vi "log analysis_gps.vi"() -> ()   [LabVIEW 2018] (continued)
126.72084266483,9.8311,22.3000,-0.0007,0.0064,0.0053,-0.805322808,0.199332071,80.524990625,0.2793,0.1938,0.4090,0.0347,0.0344,0.0317,0.0721,0.0737,4.9673,0f000005,0*f499bec4\n\tsystem status\texception 0 27.800000 0 32\trobot status\t0.669629\t-3.246177\t9.831100\t-0.805323\t0.199332\t9.475009\t0.147000\t0.222000\n\t\n15:54:09.0\tlog_raw\tgps_raw\t#INSPVAXA,USB3,0,45.0,FINESTEERING,2107,284067.050,02000000,471d,15824;INS_ALIGNMENT_COMPLETE,INS_RTKFIXED,37.37010094387,126.72084267852,9.8307,22.3000,-0.0007,0.0065,0.0059,-0.804077571,0.201412948,80.525848539,0.2693,0.1873,0.3960,0.0346,0.0343,0.0314,0.0722,0.0736,4.9532,0f000005,0*b106a646\n\tsystem status\texception 0 27.800000 0 32\trobot status\t0.670842\t-3.246592\t9.830700\t-0.804078\t0.201413\t9.474151\t0.147000\t0.222000\n\t\n15:54:09.5\tlog_raw\tgps_raw\t\tsystem status\texception 0 27.800000 0 32\trobot status\t0.671565\t-3.247256\t9.830100\t-0.803361\t0.201716\t9.474638\t0.147000\t0.222000\n\t\n15:54:10.0\tlog_raw\tgps_raw\t#INSPVAXA,USB3,0,45.0,FINESTEERING,2107,284068.050,02000000,471d,15824;INS_ALIGNMENT_COMPLETE,INS_RTKFIXED,37.37010093147,126.72084269859,9.8300,22.3000,-0.0011,0.0054,0.0061,-0.802134558,0.201672823,80.524962469,0.2605,0.1821,0.3846,0.0346,0.0343,0.0313,0.0723,0.0734,4.9387,0f000005,0*023ab06f\n\tsystem status\texception 0 27.800000 0 32\trobot status\t0.672620\t-3.247969\t9.830000\t-0.802135\t0.201673\t9.475038\t0.147000\t0.222000\n\t\n15:54:10.5\tlog_raw\tgps_raw\t\tsystem status\texception 0 27.800000 0 32\trobot status\t0.673184\t-3.248426\t9.829300\t-0.800656\t0.202458\t9.475344\t0.147000\t0.222000\n\t\n15:54:11.0\tlog_raw\tgps_raw\t\tsystem status\texception 0 27.800000 0 32\trobot status\t0.674167\t-3.248973\t9.829300\t-0.799789\t0.203840\t9.478232\t0.147000\t0.222000\n\t\n15:54:11.5\tlog_raw\tgps_raw\t#INSPVAXA,USB3,0,52.5,FINESTEERING,2107,284069.550,02000000,471d,15824;INS_ALIGNMENT_COMPLETE,INS_RTKFIXED,37.37010092244,126.72084272464,9.8293,22.3000,-0.0013,0.0057,0.0059,-0.798598974,0.203976276,80.516419675,0.2537,0.1782,0.3747,0.0345,0.0343,0.0313,0.0723,0.0733,4.9257,0f000005,0*56198093\n\tsystem status\texception 0 27.700000 0 32\trobot status\t0.674927\t-3.248971\t9.829300\t-0.798599\t0.203976\t9.483580\t0.147000\t0.222000\n\t\n15:54:12.0\tlog_raw\tgps_raw\t#INSPVAXA,USB3,0,52.5,FINESTEERING,2107,284070.050,02000000,471d,15824;INS_ALIGNMENT_COMPLETE,INS_RTKFIXED,37.37010091982,126.72084273744,9.8297,22.3000,-0.0012,0.0080,0.0052,-0.796727291,0.202371402,80.509450854,0.2478,0.1752,0.3659,0.0345,0.0343,0.0313,0.0724,0.0732,4.9128,0f000005,0*32eb7788\n\tsystem status\texception 0 27.800000 0 32\trobot status\t0.676061\t-3.249262\t9.829700\t-0.796727\t0.202371\t9.490549\t0.147000\t0.222000\n\t\n15:54:12.5\tlog_raw\tgps_raw\t\tsystem status\texception 0 27.800000 0 32\trobot status\t0.674655\t-3.249824\t9.829400\t-0.792783\t0.205130\t9.497173\t0.147000\t0.222000\n\t\n15:54:13.0\tlog_raw\tgps_raw\t#INSPVAXA,USB3,0,48.5,FINESTEERING,2107,284071.050,02000000,471d,15824;INS_ALIGNMENT_COMPLETE,INS_RTKFIXED,37.37010090434,126.72084271110,9.8295,22.3000,-0.0039,0.0026,0.0058,-0.794464008,0.206738241,80.502187928,0.2427,0.1727,0.3579,0.0345,0.0343,0.0313,0.0724,0.0732,4.9038,0f000005,0*ae7eb45b\n\tsystem status\texception 0 27.800000 0 32\trobot status\t0.673728\t-3.250980\t9.829500\t-0.794464\t0.206738\t9.497812\t0.147000\t0.222000\n\t\n15:54:13.5\tlog_raw\tgps_raw\t#INSPVAXA,USB3,0,48.5,FINESTEERING,2107,284071.550,02000000,471d,15824;INS_ALIGNMENT_COMPLETE,INS_RTKFIXED,37.37010089734,126.72084271003,9.8294,22.3000,-0.0047,0.0026,0.0048,-0.792309552,0.204330401,80.495522274,0.2427,0.1727,0.3579,0.0345,0.0343,0.0313,0.0724,0.0732,4.9038,0f000005,0*ad98db8e\n\tsystem status\texception 0 27.800000 0 32\trobot status\t0.673633\t-3.251756\t9.829400\t-0.792310\t0.204330\t9.504478\t0.147000\t0.222000\n\t\n15:54:14.0\tlog_raw\tgps_raw\t\tsystem status\texception 0 27.800000 0 32\trobot status\t0.673376\t-3.253810\t9.829800\t-0.795967\t0.184821\t9.359598\t0.117000\t0.095000\n\t\n15:54:14.5\tlog_raw\tgps_raw\t\tsystem status\texception 0 27.800000 0 60\trobot status\t0.674132\t-3.257605\t9.832900\t-0.788414\t0.193198\t9.387077\t0.117000\t0.095000\n\t\n15:54:15.0\tlog_raw\tgps_raw\t\tsystem status\texception 0 27.800000 0 60\trobot status\t0.676499\t-3.262353\t9.836500\t-0.786147\t0.194904\t9.385323\t0.117000\t0.095000\n\t\n15:54:15.5\tlog_raw\tgps_raw\t\tsystem status\texception 0 27.800000 0 60\trobot status\t0.678961\t-3.267673\t9.840700\t-0.786580\t0.194426\t9.385900\t0.117000\t0.095000\n\t\n15:54:16.0\tlog_raw\tgps_raw\t\tsystem status\texception 0 27.800000 0 60\trobot status\t0.682045\t-3.274174\t9.845300\t-0.785139\t0.194086\t9.384595\t0.117000\t0.095000\n\t\n15:54:16.5\tlog_raw\tgps_raw\t\tsystem status\texception 0 27.800000 0 60\trobot status\t0.684298\t-3.281012\t9.849500\t-0.785110\t0.192293\t9.376254\t0.117000\t0.095000\n\t\n15:54:17.0\tlog_raw\tgps_raw\t\tsystem status\texception 0 27.800000 0 60\trobot status\t0.687811\t-3.288802\t9.854200\t-0.783660\t0.192337\t9.377009\t0.117000\t0.095000\n\t\n15:54:17.5\tlog_raw\tgps_raw\t\tsystem status\texception 0 27.800000 0 60\trobot status\t0.690737\t-3.295775\t9.858800\t-0.784560\t0.190680\t9.377608\t0.117000\t0.095000\n\t\n15:54:18.0\tlog_raw\tgps_raw\t#INSPVAXA,USB3,0,53.5,FINESTEERING,2107,284076.050,02000000,471d,15824;INS_ALIGNMENT_COMPLETE,INS_RTKFIXED,37.37010043153,126.72084293702,9.8639,22.3000,-0.0224,0.0084,0.0124,-0.782520442,0.190697298,80.620510756,0.3079,0.2467,0.3912,0.0928,0.0849,0.0629,0.0895,0.0915,4.9091,0f000001,0*151fdb37\n\tsystem status\texception 0 27.800000 0 60\trobot status\t0.693740\t-3.303454\t9.863900\t-0.782520\t0.190697\t9.379489\t0.117000\t0.095000\n\t\n15:54:18.5\tlog_raw\tgps_raw\t\tsystem status\texception 0 27.800000 0 60\trobot status\t0.697678\t-3.308999\t9.869500\t-0.783353\t0.190598\t9.384457\t0.117000\t0.095000\n\t\n15:54:19.0\tlog_raw\tgps_raw\t\tsystem status\texception 0 27.800000 0 60\trobot status\t0.701548\t-3.315091\t9.875400\t-0.783389\t0.191366\t9.388017\t0.117000\t0.095000\n\t\n15:54:19.5\tlog_raw\tgps_raw\t#INSPVAXA,USB3,0,53.0,FINESTEERING,2107,284077.550,02000000,471d,15824;INS_ALIGNMENT_COMPLETE,INS_RTKFIXED,37.37010029205,126.72084303769,9.8807,22.3000,-0.0245,0.0085,0.0134,-0.783196665,0.189878552,80.605229248,0.3387,0.2662,0.4111,0.1003,0.0889,0.0668,0.0907,0.0935,4.9083,0f000001,0*a805bdc6\n\tsystem status\texception 0 27.800000 0 60\trobot status\t0.702657\t-3.318934\t9.880700\t-0.783197\t0.189879\t9.394771\t0.117000\t0.095000\n\t\n15:54:20.0\tlog_raw\tgps_raw\t\t", "INSPVAXA,USB3,0,52.0,FINESTEERING,2107,284098.100,02000000,471d,15824;INS_ALIGNMENT_COMPLETE,INS_RTKFIXED,37.37010081715,126.72084280567,9.8392,22.3000,-0.0127,0.0026,0.0011,-0.779185291,0.204850370,80.324830339,0.2135,0.1621,0.2919,0.0344,0.0343,0.0312,0.0727,0.0733,4.8847,0f000005,0*b965a086\n\t", "INSPVAXA,USB3,0,53.0,FINESTEERING,2107,284099.100,02000000,471d,15824;INS_ALIGNMENT_COMPLETE,INS_RTKFIXED,37.37010080039,126.72084280580,9.8388,22.3000,-0.0144,0.0013,0.0007,-0.778559962,0.207012458,80.310324133,0.2130,0.1619,0.2904,0.0344,0.0343,0.0312,0.0727,0.0733,4.8855,0f000005,0*91b9a8e7\n\t", "INSPVAXA,USB3,0,50.0,FINESTEERING,2107,284101.100,02000000,471d,15824;INS_ALIGNMENT_COMPLETE,INS_RTKFIXED,37.37010080256,126.72084279427,9.8376,22.3000,-0.0100,0.0003,0.0004,-0.784971071,0.210053203,80.284000785,0.2120,0.1618,0.2876,0.0344,0.0343,0.0312,0.0727,0.0733,4.8873,0f000005,0*ce207b7d\n\t", "INSPVAXA,USB3,0,50.0,FINESTEERING,2107,284101.600,02000000,471d,15824;INS_ALIGNMENT_COMPLETE,INS_RTKFIXED,37.37010080771,126.72084279588,9.8375,22.3000,-0.0097,0.0008,0.0002,-0.787245577,0.212021074,80.277840242,0.2120,0.1618,0.2876,0.0344,0.0343,0.0312,0.0727,0.0733,4.8873,0f000005,0*d3394abe\n\t", "INSPVAXA,USB3,0,53.0,FINESTEERING,2107,284102.100,02000000,471d,15824;INS_ALIGNMENT_COMPLETE,INS_RTKFIXED,37.37010080827,126.72084279791,9.8372,22.3000,-0.0086,0.0007,-0.0005,-0.787222200,0.211318071,80.272885297,0.2116,0.1617,0.2864,0.0344,0.0343,0.0312,0.0727,0.0733,4.8883,0f000005,0*7e8ab6e8\n\t", "INSPVAXA,USB3,0,53.0,FINESTEERING,2107,284103.100,02000000,471d,15824;INS_ALIGNMENT_COMPLETE,INS_RTKFIXED,37.37010082403,126.72084278484,9.8365,22.3000,-0.0064,-0.0008,-0.0001,-0.787428816,0.215864037,80.263823554,0.2112,0.1616,0.2853,0.0344,0.0343,0.0312,0.0727,0.0733,4.8894,0f000005,0*f475c441\n\t", "INSPVAXA,USB3,0,53.0,FINESTEERING,2107,284104.050,02000000,471d,15824;INS_ALIGNMENT_COMPLETE,INS_RTKFIXED,37.37010082408,126.72084278410,9.8363,22.3000,-0.0077,0.0002,0.0002,-0.786930858,0.220983047,80.255496235,0.2109,0.1616,0.2842,0.0344,0.0343,0.0312,0.0727,0.0733,4.8905,0f000005,0*84218c18\n\t", "INSPVAXA,USB3,0,53.0,FINESTEERING,2107,284104.050,02000000,471d,15824;INS_ALIGNMENT_COMPLETE,INS_RTKFIXED,37.37010082408,126.72084278410,9.8363,22.3000,-0.0077,0.0002,0.0002,-0.786930858,0.220983047,80.255496235,0.2109,0.1616,0.2842,0.0344,0.0343,0.0312,0.0727,0.0733,4.8905,0f000005,0*84218c18\n\t", "INSPVAXA,USB3,0,53.0,FINESTEERING,2107,284104.050,02000000,471d,15824;INS_ALIGNMENT_COMPLETE,INS_RTKFIXED,37.37010082408,126.72084278410,9.8363,22.3000,-0.0077,0.0002,0.0002,-0.786930858,0.220983047,80.255496235,0.2109,0.1616,0.2842,0.0344,0.0343,0.0312,0.0727,0.0733,4.8905,0f000005,0*84218c18\n\t", "INSPVAXA,USB3,0,53.0,FINESTEERING,2107,284104.050,02000000,471d,15824;INS_ALIGNMENT_COMPLETE,INS_RTKFIXED,37.37010082408,126.72084278410,9.8363,22.3000,-0.0077,0.0002,0.0002,-0.786930858,0.220983047,80.255496235,0.2109,0.1616,0.2842,0.0344,0.0343,0.0312,0.0727,0.0733,4.8905,0f000005,0*84218c18\n\t", "INSPVAXA,USB3,0,53.0,FINESTEERING,2107,284104.050,02000000,471d,15824;INS_ALIGNMENT_COMPLETE,INS_RTKFIXED,37.37010082408,126.72084278410,9.8363,22.3000,-0.0077,0.0002,0.0002,-0.786930858,0.220983047,80.255496235,0.2109,0.1616,0.2842,0.0344,0.0343,0.0312,0.0727,0.0733,4.8905,0f000005,0*84218c18\n\t", "INSPVAXA,USB3,0,53.0,FINESTEERING,2107,284104.050,02000000,471d,15824;INS_ALIGNMENT_COMPLETE,INS_RTKFIXED,37.37010082408,126.72084278410,9.8363,22.3000,-0.0077,0.0002,0.0002,-0.786930858,0.220983047,80.255496235,0.2109,0.1616,0.2842,0.0344,0.0343,0.0312,0.0727,0.0733,4.8905,0f000005,0*84218c18\n\t", "INSPVAXA,USB3,0,53.0,FINESTEERING,2107,284104.050,02000000,471d,15824;INS_ALIGNMENT_COMPLETE,INS_RTKFIXED,37.37010082408,126.72084278410,9.8363,22.3000,-0.0077,0.0002,0.0002,-0.786930858,0.220983047,80.255496235,0.2109,0.1616,0.2842,0.0344,0.0343,0.0312,0.0727,0.0733,4.8905,0f000005,0*84218c18\n\t", "INSPVAXA,USB3,0,53.0,FINESTEERING,2107,284104.050,02000000,471d,15824;INS_ALIGNMENT_COMPLETE,INS_RTKFIXED,37.37010082408,126.72084278410,9.8363,22.3000,-0.0077,0.0002,0.0002,-0.786930858,0.220983047,80.255496235,0.2109,0.1616,0.2842,0.0344,0.0343,0.0312,0.0727,0.0733,4.8905,0f000005,0*84218c18\n\t", "INSPVAXA,USB3,0,53.0,FINESTEERING,2107,284104.050,02000000,471d,15824;INS_ALIGNMENT_COMPLETE,INS_RTKFIXED,37.37010082408,126.72084278410,9.8363,22.3000,-0.0077,0.0002,0.0002,-0.786930858,0.220983047,80.255496235,0.2109,0.1616,0.2842,0.0344,0.0343,0.0312,0.0727,0.0733,4.8905,0f000005,0*84218c18\n\t", "INSPVAXA,USB3,0,53.0,FINESTEERING,2107,284104.050,02000000,471d,15824;INS_ALIGNMENT_COMPLETE,INS_RTKFIXED,37.37010082408,126.72084278410,9.8363,22.3000,-0.0077,0.0002,0.0002,-0.786930858,0.220983047,80.255496235,0.2109,0.1616,0.2842,0.0344,0.0343,0.0312,0.0727,0.0733,4.8905,0f000005,0*84218c18\n\t", "INSPVAXA,USB3,0,53.0,FINESTEERING,2107,284104.050,02000000,471d,15824;INS_ALIGNMENT_COMPLETE,INS_RTKFIXED,37.37010082408,126.72084278410,9.8363,22.3000,-0.0077,0.0002,0.0002,-0.786930858,0.220983047,80.255496235,0.2109,0.1616,0.2842,0.0344,0.0343,0.0312,0.0727,0.0733,4.8905,0f000005,0*84218c18\n\t", "INSPVAXA,USB3,0,53.0,FINESTEERING,2107,284104.050,02000000,471d,15824;INS_ALIGNMENT_COMPLETE,INS_RTKFIXED,37.37010082408,126.72084278410,9.8363,22.3000,-0.0077,0.0002,0.0002,-0.786930858,0.220983047,80.255496235,0.2109,0.1616,0.2842,0.0344,0.0343,0.0312,0.0727,0.0733,4.8905,0f000005,0*84218c18\n\t", "INSPVAXA,USB3,0,53.0,FINESTEERING,2107,284104.050,02000000,471d,15824;INS_ALIGNMENT_COMPLETE,INS_RTKFIXED,37.37010082408,126.72084278410,9.8363,22.3000,-0.0077,0.0002,0.0002,-0.786930858,0.220983047,80.255496235,0.2109,0.1616,0.2842,0.0344,0.0343,0.0312,0.0727,0.0733,4.8905,0f000005,0*84218c18\n\t", "INSPVAXA,USB3,0,53.0,FINESTEERING,2107,284104.050,02000000,471d,15824;INS_ALIGNMENT_COMPLETE,INS_RTKFIXED,37.37010082408,126.72084278410,9.8363,22.3000,-0.0077,0.0002,0.0002,-0.786930858,0.220983047,80.255496235,0.2109,0.1616,0.2842,0.0344,0.0343,0.0312,0.0727,0.0733,4.8905,0f000005,0*84218c18\n\t", "INSPVAXA,USB3,0,53.0,FINESTEERING,2107,284104.050,02000000,471d,15824;INS_ALIGNMENT_COMPLETE,INS_RTKFIXED,37.37010082408,126.72084278410,9.8363,22.3000,-0.0077,0.0002,0.0002,-0.786930858,0.220983047,80.255496235,0.2109,0.1616,0.2842,0.0344,0.0343,0.0312,0.0727,0.0733,4.8905,0f000005,0*84218c18\n\t", "INSPVAXA,USB3,0,53.0,FINESTEERING,2107,284104.050,02000000,471d,15824;INS_ALIGNMENT_COMPLETE,INS_RTKFIXED,37.37010082408,126.72084278410,9.8363,22.3000,-0.0077,0.0002,0.0002,-0.786930858,0.220983047,80.255496235,0.2109,0.1616,0.2842,0.0344,0.0343,0.0312,0.0727,0.0733,4.8905,0f000005,0*84218c18\n\t", "INSPVAXA,USB3,0,53.0,FINESTEERING,2107,284104.050,02000000,471d,15824;INS_ALIGNMENT_COMPLETE,INS_RTKFIXED,37.37010082408,126.72084278410,9.8363,22.3000,-0.0077,0.0002,0.0002,-0.786930858,0.220983047,80.255496235,0.2109,0.1616,0.2842,0.0344,0.0343,0.0312,0.0727,0.0733,4.8905,0f000005,0*84218c18\n\t", "INSPVAXA,USB3,0,53.0,FINESTEERING,2107,284104.050,02000000,471d,15824;INS_ALIGNMENT_COMPLETE,INS_RTKFIXED,37.37010082408,126.72084278410,9.8363,22.3000,-0.0077,0.0002,0.0002,-0.786930858,0.220983047,80.255496235,0.2109,0.1616,0.2842,0.0344,0.0343,0.0312,0.0727,0.0733,4.8905,0f000005,0*84218c18\n\t", "INSPVAXA,USB3,0,53.0,FINESTEERING,2107,284104.050,02000000,471d,15824;INS_ALIGNMENT_COMPLETE,INS_RTKFIXED,37.37010082408,126.72084278410,9.8363,22.3000,-0.0077,0.0002,0.0002,-0.786930858,0.220983047,80.255496235,0.2109,0.1616,0.2842,0.0344,0.0343,0.0312,0.0727,0.0733,4.8905,0f000005,0*84218c18\n\t", "INSPVAXA,USB3,0,53.0,FINESTEERING,2107,284104.050,02000000,471d,15824;INS_ALIGNMENT_COMPLETE,INS_RTKFIXED,37.37010082408,126.72084278410,9.8363,22.3000,-0.0077,0.0002,0.0002,-0.786930858,0.220983047,80.255496235,0.2109,0.1616,0.2842,0.0344,0.0343,0.0312,0.0727,0.0733,4.8905,0f000005,0*84218c18\n\t", "INSPVAXA,USB3,0,53.0,FINESTEERING,2107,284104.050,02000000,471d,15824;INS_ALIGNMENT_COMPLETE,INS_RTKFIXED,37.37010082408,126.72084278410,9.8363,22.3000,-0.0077,0.0002,0.0002,-0.786930858,0.220983047,80.255496235,0.2109,0.1616,0.2842,0.0344,0.0343,0.0312,0.0727,0.0733,4.8905,0f000005,0*84218c18\n\t", "INSPVAXA,USB3,0,53.0,FINESTEERING,2107,284104.050,02000000,471d,15824;INS_ALIGNMENT_COMPLETE,INS_RTKFIXED,37.37010082408,126.72084278410,9.8363,22.3000,-0.0077,0.0002,0.0002,-0.786930858,0.220983047,80.255496235,0.2109,0.1616,0.2842,0.0344,0.0343,0.0312,0.0727,0.0733,4.8905,0f000005,0*84218c18\n\t", "INSPVAXA,USB3,0,53.0,FINESTEERING,2107,284104.050,02000000,471d,15824;INS_ALIGNMENT_COMPLETE,INS_RTKFIXED,37.37010082408,126.72084278410,9.8363,22.3000,-0.0077,0.0002,0.0002,-0.786930858,0.220983047,80.255496235,0.2109,0.1616,0.2842,0.0344,0.0343,0.0312,0.0727,0.0733,4.8905,0f000005,0*84218c18\n\t", "INSPVAXA,USB3,0,53.0,FINESTEERING,2107,284104.050,02000000,471d,15824;INS_ALIGNMENT_COMPLETE,INS_RTKFIXED,37.37010082408,126.72084278410,9.8363,22.3000,-0.0077,0.0002,0.0002,-0.786930858,0.220983047,80.255496235,0.2109,0.1616,0.2842,0.0344,0.0343,0.0312,0.0727,0.0733,4.8905,0f000005,0*84218c18\n\t", "INSPVAXA,USB3,0,53.0,FINESTEERING,2107,284104.050,02000000,471d,15824;INS_ALIGNMENT_COMPLETE,INS_RTKFIXED,37.37010082408,126.72084278410,9.8363,22.3000,-0.0077,0.0002,0.0002,-0.786930858,0.220983047,80.255496235,0.2109,0.1616,0.2842,0.0344,0.0343,0.0312,0.0727,0.0733,4.8905,0f000005,0*84218c18\n\t", "INSPVAXA,USB3,0,53.0,FINESTEERING,2107,284104.050,02000000,471d,15824;INS_ALIGNMENT_COMPLETE,INS_RTKFIXED,37.37010082408,126.72084278410,9.8363,22.3000,-0.0077,0.0002,0.0002,-0.786930858,0.220983047,80.255496235,0.2109,0.1616,0.2842,0.0344,0.0343,0.0312,0.0727,0.0733,4.8905,0f000005,0*84218c18\n\t", "INSPVAXA,USB3,0,53.0,FINESTEERING,2107,284104.050,02000000,471d,15824;INS_ALIGNMENT_COMPLETE,INS_RTKFIXED,37.37010082408,126.72084278410,9.8363,22.3000,-0.0077,0.0002,0.0002,-0.786930858,0.220983047,80.255496235,0.2109,0.1616,0.2842,0.0344,0.0343,0.0312,0.0727,0.0733,4.8905,0f000005,0*84218c18\n\t", "INSPVAXA,USB3,0,53.0,FINESTEERING,2107,284104.050,02000000,471d,15824;INS_ALIGNMENT_COMPLETE,INS_RTKFIXED,37.37010082408,126.72084278410,9.8363,22.3000,-0.0077,0.0002,0.0002,-0.786930858,0.220983047,80.255496235,0.2109,0.1616,0.2842,0.0344,0.0343,0.0312,0.0727,0.0733,4.8905,0f000005,0*84218c18\n\t", "INSPVAXA,USB3,0,53.0,FINESTEERING,2107,284104.050,02000000,471d,15824;INS_ALIGNMENT_COMPLETE,INS_RTKFIXED,37.37010082408,126.72084278410,9.8363,22.3000,-0.0077,0.0002,0.0002,-0.786930858,0.220983047,80.255496235,0.2109,0.1616,0.2842,0.0344,0.0343,0.0312,0.0727,0.0733,4.8905,0f000005,0*84218c18\n\t", "INSPVAXA,USB3,0,53.0,FINESTEERING,2107,284104.050,02000000,471d,15824;INS_ALIGNMENT_COMPLETE,INS_RTKFIXED,37.37010082408,126.72084278410,9.8363,22.3000,-0.0077,0.0002,0.0002,-0.786930858,0.220983047,80.255496235,0.2109,0.1616,0.2842,0.0344,0.0343,0.0312,0.0727,0.0733,4.8905,0f000005,0*84218c18\n\t", "INSPVAXA,USB3,0,53.0,FINESTEERING,2107,284104.050,02000000,471d,15824;INS_ALIGNMENT_COMPLETE,INS_RTKFIXED,37.37010082408,126.72084278410,9.8363,22.3000,-0.0077,0.0002,0.0002,-0.786930858,0.220983047,80.255496235,0.2109,0.1616,0.2842,0.0344,0.0343,0.0312,0.0727,0.0733,4.8905,0f000005,0*84218c18\n\t", "INSPVAXA,USB3,0,53.0,FINESTEERING,2107,284104.050,02000000,471d,15824;INS_ALIGNMENT_COMPLETE,INS_RTKFIXED,37.37010082408,126.72084278410,9.8363,22.3000,-0.0077,0.0002,0.0002,-0.786930858,0.220983047,80.255496235,0.2109,0.1616,0.2842,0.0344,0.0343,0.0312,0.0727,0.0733,4.8905,0f000005,0*84218c18\n\t", "INSPVAXA,USB3,0,53.0,FINESTEERING,2107,284104.050,02000000,471d,15824;INS_ALIGNMENT_COMPLETE,INS_RTKFIXED,37.37010082408,126.72084278410,9.8363,22.3000,-0.0077,0.0002,0.0002,-0.786930858,0.220983047,80.255496235,0.2109,0.1616,0.2842,0.0344,0.0343,0.0312,0.0727,0.0733,4.8905,0f000005,0*84218c18\n\t", "INSPVAXA,USB3,0,53.0,FINESTEERING,2107,284104.050,02000000,471d,15824;INS_ALIGNMENT_COMPLETE,INS_RTKFIXED,37.37010082408,126.72084278410,9.8363,22.3000,-0.0077,0.0002,0.0002,-0.786930858,0.220983047,80.255496235,0.2109,0.1616,0.2842,0.0344,0.0343,0.0312,0.0727,0.0733,4.8905,0f000005,0*84218c18\n\t", "INSPVAXA,USB3,0,53.0,FINESTEERING,2107,284104.050,02000000,471d,15824;INS_ALIGNMENT_COMPLETE,INS_RTKFIXED,37.37010082408,126.72084278410,9.8363,22.3000,-0.0077,0.0002,0.0002,-0.786930858,0.220983047,80.255496235,0.2109,0.1616,0.2842,0.0344,0.0343,0.0312,0.0727,0.0733,4.8905,0f000005,0*84218c18\n\t", "INSPVAXA,USB3,0,53.0,FINESTEERING,2107,284104.050,02000000,471d,15824;INS_ALIGNMENT_COMPLETE,INS_RTKFIXED,37.37010082408,126.72084278410,9.8363,22.3000,-0.0077,0.0002,0.0002,-0.786930858,0.220983047,80.255496235,0.2109,0.1616,0.2842,0.0344,0.0343,0.0312,0.0727,0.0733,4.8905,0f000005,0*84218c18\n\t", "INSPVAXA,USB3,0,53.0,FINESTEERING,2107,284104.050,02000000,471d,15824;INS_ALIGNMENT_COMPLETE,INS_RTKFIXED,37.37010082408,126.72084278410,9.8363,22.3000,-0.0077,0.0002,0.0002,-0.786930858,0.220983047,80.255496235,0.2109,0.1616,0.2842,0.0344,0.0343,0.0312,0.0727,0.0733,4.8905,0f000005,0*84218c18\n\t", "INSPVAXA,USB3,0,53.0,FINESTEERING,2107,284104.050,02000000,471d,15824;INS_ALIGNMENT_COMPLETE,INS_RTKFIXED,37.37010082408,126.72084278410,9.8363,22.3000,-0.0077,0.0002,0.0002,-0.786930858,0.220983047,80.255496235,0.2109,0.1616,0.2842,0.0344,0.0343,0.0312,0.0727,0.0733,4.8905,0f000005,0*84218c18\n\t", "INSPVAXA,USB3,0,53.0,FINESTEERING,2107,284104.050,02000000,471d,15824;INS_ALIGNMENT_COMPLETE,INS_RTKFIXED,37.37010082408,126.72084278410,9.8363,22.3000,-0.0077,0.0002,0.0002,-0.786930858,0.220983047,80.255496235,0.2109,0.1616,0.2842,0.0344,0.0343,0.0312,0.0727,0.0733,4.8905,0f000005,0*84218c18\n\t", "INSPVAXA,USB3,0,53.0,FINESTEERING,2107,284104.050,02000000,471d,15824;INS_ALIGNMENT_COMPLETE,INS_RTKFIXED,37.37010082408,126.72084278410,9.8363,22.3000,-0.0077,0.0002,0.0002,-0.786930858,0.220983047,80.255496235,0.2109,0.1616,0.2842,0.0344,0.0343,0.0312,0.0727,0.0733,4.8905,0f000005,0*84218c18\n\t", "INSPVAXA,USB3,0,53.0,FINESTEERING,2107,284104.050,02000000,471d,15824;INS_ALIGNMENT_COMPLETE,INS_RTKFIXED,37.37010082408,126.72084278410,9.8363,22.3000,-0.0077,0.0002,0.0002,-0.786930858,0.220983047,80.255496235,0.2109,0.1616,0.2842,0.0344,0.0343,0.0312,0.0727,0.0733,4.8905,0f000005,0*84218c18\n\t", "INSPVAXA,USB3,0,53.0,FINESTEERING,2107,284104.050,02000000,471d,15824;INS_ALIGNMENT_COMPLETE,INS_RTKFIXED,37.37010082408,126.72084278410,9.8363,22.3000,-0.0077,0.0002,0.0002,-0.786930858,0.220983047,80.255496235,0.2109,0.1616,0.2842,0.0344,0.0343,0.0312,0.0727,0.0733,4.8905,0f000005,0*84218c18\n\t", "INSPVAXA,USB3,0,53.0,FINESTEERING,2107,284104.050,02000000,471d,15824;INS_ALIGNMENT_COMPLETE,INS_RTKFIXED,37.37010082408,126.72084278410,9.8363,22.3000,-0.0077,0.0002,0.0002,-0.786930858,0.220983047,80.255496235,0.2109,0.1616,0.2842,0.0344,0.0343,0.0312,0.0727,0.0733,4.8905,0f000005,0*84218c18\n\t", "INSPVAXA,USB3,0,53.0,FINESTEERING,2107,284104.050,02000000,471d,15824;INS_ALIGNMENT_COMPLETE,INS_RTKFIXED,37.37010082408,126.72084278410,9.8363,22.3000,-0.0077,0.0002,0.0002,-0.786930858,0.220983047,80.255496235,0.2109,0.1616,0.2842,0.0344,0.0343,0.0312,0.0727,0.0733,4.8905,0f000005,0*84218c18\n\t", "INSPVAXA,USB3,0,53.0,FINESTEERING,2107,284104.050,02000000,471d,15824;INS_ALIGNMENT_COMPLETE,INS_RTKFIXED,37.37010082408,126.72084278410,9.8363,22.3000,-0.0077,0.0002,0.0002,-0.786930858,0.220983047,80.255496235,0.2109,0.1616,0.2842,0.0344,0.0343,0.0312,0.0727,0.0733,4.8905,0f000005,0*84218c18\n\t", "INSPVAXA,USB3,0,53.0,FINESTEERING,2107,284104.050,02000000,471d,15824;INS_ALIGNMENT_COMPLETE,INS_RTKFIXED,37.37010082408,126.72084278410,9.8363,22.3000,-0.0077,0.0002,0.0002,-0.786930858,0.220983047,80.255496235,0.2109,0.1616,0.2842,0.0344,0.0343,0.0312,0.0727,0.0733,4.8905,0f000005,0*84218c18\n\t", "INSPVAXA,USB3,0,53.0,FINESTEERING,2107,284104.050,02000000,471d,15824;INS_ALIGNMENT_COMPLETE,INS_RTKFIXED,37.37010082408,126.72084278410,9.8363,22.3000,-0.0077,0.0002,0.0002,-0.786930858,0.220983047,80.255496235,0.2109,0.1616,0.2842,0.0344,0.0343,0.0312,0.0727,0.0733,4.8905,0f000005,0*84218c18\n\t", "INSPVAXA,USB3,0,53.0,FINESTEERING,2107,284104.050,02000000,471d,15824;INS_ALIGNMENT_COMPLETE,INS_RTKFIXED,37.37010082408,126.72084278410,9.8363,22.3000,-0.0077,0.0002,0.0002,-0.786930858,0.220983047,80.255496235,0.2109,0.1616,0.2842,0.0344,0.0343,0.0312,0.0727,0.0733,4.8905,0f000005,0*84218c18\n\t", "INSPVAXA,USB3,0,53.0,FINESTEERING,2107,284104.050,02000000,471d,15824;INS_ALIGNMENT_COMPLETE,INS_RTKFIXED,37.37010082408,126.72084278410,9.8363,22.3000,-0.0077,0.0002,0.0002,-0.786930858,0.220983047,80.255496235,0.2109,0.1616,0.2842,0.0344,0.0343,0.0312,0.0727,0.0733,4.8905,0f000005,0*84218c18\n\t", "INSPVAXA,USB3,0,53.0,FINESTEERING,2107,284104.050,02000000,471d,15824;INS_ALIGNMENT_COMPLETE,INS_RTKFIXED,37.37010082408,126.72084278410,9.8363,22.3000,-0.0077,0.0002,0.0002,-0.786930858,0.220983047,80.255496235,0.2109,0.1616,0.2842,0.0344,0.0343,0.0312,0.0727,0.0733,4.8905,0f000005,0*84218c18\n\t", ""]
  out "이전 부분 문자열":string
  in  "load":bool
  in  "path":path=path "C:/Users/WeGo/Desktop/patrol robot/log/patrol-0527_log.txt"
  out "텍스트":string="15:04:55.6\tlog_raw\tgps_raw\t\tsystem status\tnormal 0 28.400000 0 0\trobot status\t0.573944\t0.974098\t9.870700\t-0.040116\t-0.068991\t52.206776\t0.000000\t-0.001000\n\t\n15:04:56.1\tlog_raw\tgps_raw\t\tsystem status\tnormal 0 28.400000 0 0\trobot status\t0.573944\t0.974098\t9.870700\t-0.040116\t-0.068991\t52.206776\t0.000000\t-0.001000\n\t\n15:04:56.6\tlog_raw\tgps_raw\t\tsystem status\tnormal 0 28.400000 0 0\trobot status\t0.573944\t0.974098\t9.870700\t-0.040116\t-0.068991\t52.206776\t0.000000\t-0.001000\n\t\n15:04:57.1\tlog_raw\tgps_raw\t\tsystem status\tnormal 0 28.400000 0 0\trobot status\t0.573944\t0.974098\t9.870700\t-0.040116\t-0.068991\t52.206776\t0.000000\t-0.001000\n\t\n15:04:57.6\tlog_raw\tgps_raw\t\tsystem status\tnormal 0 28.400000 0 0\trobot status\t0.573944\t0.974098\t9.870700\t-0.040116\t-0.068991\t52.206776\t0.000000\t-0.001000\n\t\n15:04:58.1\tlog_raw\tgps_raw\t\tsystem status\tnormal 0 28.400000 0 0\trobot status\t0.573944\t0.974098\t9.870700\t-0.040116\t-0.068991\t52.206776\t0.000000\t-0.001000\n\t\n15:04:58.6\tlog_raw\tgps_raw\t\tsystem status\tnormal 0 28.300000 0 0\trobot status\t0.573944\t0.974098\t9.870700\t-0.040116\t-0.068991\t52.206776\t0.000000\t-0.001000\n\t\n15:04:59.1\tlog_raw\tgps_raw\t\tsystem status\tnormal 0 28.400000 0 0\trobot status\t0.573944\t0.974098\t9.870700\t-0.040116\t-0.068991\t52.206776\t0.000000\t-0.001000\n\t\n15:04:59.6\tlog_raw\tgps_raw\t\tsystem status\tnormal 0 28.400000 0 0\trobot status\t0.573944\t0.974098\t9.870700\t-0.040116\t-0.068991\t52.206776\t0.000000\t-0.001000\n\t\n15:05:00.1\tlog_raw\tgps_raw\t#INSPVAXA,USB3,0,51.0,FINESTEERING,2107,281115.600,02000000,471d,15824;INS_ALIGNMENT_COMPLETE,INS_RTKFIXED,37.37013888668,126.72084169564,9.8834,22.3000,0.0026,0.0071,0.0017,-0.044376618,-0.064379115,35.875304095,0.1980,0.1670,0.2645,0.0373,0.0373,0.0312,0.3280,0.3375,5.4270,0f000015,0*6411398e\n\tsystem status\tnormal 0 28.400000 0 0\trobot status\t0.583780\t0.964475\t9.883400\t-0.044377\t-0.064379\t52.206776\t0.000000\t-0.001000\n\t\n15:05:00.6\tlog_raw\tgps_raw\t#DUALANTENNAHEADINGA,USB3,0,47.5,FINESTEERING,2107,281116.400,02000000,d426,15824;SOL_COMPUTED,NARROW_INT,-1.000000000,37.878738403,-13.522033691,0.0,0.725115359,0.922636747,\"631T\",26,18,18,14,04,01,30,33*26208e7b\n\tsystem status\tnormal 0 28.400000 0 0\trobot status\t0.584352\t0.964624\t9.883500\t-0.048962\t-0.060425\t52.121262\t0.000000\t0.000000\n\t\n15:05:01.1\tlog_raw\tgps_raw\t#INSPVAXA,USB3,0,40.0,FINESTEERING,2107,281117.200,02000000,471d,15824;INS_ALIGNMENT_COMPLETE,INS_RTKFIXED,37.37013888274,126.72084170690,9.8836,22.3000,0.0013,0.0059,0.0019,-0.052026954,-0.057051348,35.889318154,0.1981,0.1668,0.2641,0.0380,0.0379,0.0312,0.3290,0.3384,5.4011,0f000015,0*fd51250c\n\tsystem status\tnormal 0 28.400000 0 0\trobot status\t0.584778\t0.964038\t9.883600\t-0.052027\t-0.057051\t52.074791\t0.000000\t0.000000\n\t\n15:05:01.6\tlog_raw\tgps_raw\t#INSPVAXA,USB3,0,40.0,FINESTEERING,2107,281118.000,02000000,471d,15824;INS_ALIGNMENT_COMPLETE,INS_RTKFIXED,37.37013888102,126.72084170383,9.8834,22.3000,0.0019,0.0041,0.0020,-0.055362529,-0.053444915,35.896365785,0.1981,0.1668,0.2641,0.0380,0.0379,0.0312,0.3290,0.3384,5.4011,0f000015,0*f14a9826\n\tsystem status\tnormal 0 28.400000 0 0\trobot status\t0.584506\t0.963847\t9.883400\t-0.055363\t-0.053445\t52.062977\t0.000000\t0.000000\n\t\n15:05:02.1\tlog_raw\tgps_raw\t#DUALANTENNAHEADINGA,USB3,0,44.0,FINESTEERING,2107,281118.800,02000000,d426,15824;SOL_COMPUTED,NARROW_INT,-1.000000000,37.760478973,-13.751342773,0.0,0.572546124,0.783588052,\"631T\",29,18,18,14,04,01,30,33*16eb02ed\n\tsystem status\tnormal 0 28.400000 0 0\trobot status\t0.582978\t0.963809\t9.883100\t-0.060167\t-0.049421\t52.239521\t0.000000\t-0.001000\n\t\n15:05:02.6\tlog_raw\tgps_raw\t#DUALANTENNAHEADINGA,USB3,0,43.5,FINESTEERING,2107,281119.600,02000000,d426,15824;SOL_COMPUTED,NARROW_INT,-1.000000000,37.875923157,-13.317504883,0.0,0.559661269,0.773583710,\"631T\",28,18,18,14,04,01,30,33*05407579\n\tsystem status\tnormal 0 28.300000 0 0\trobot status\t0.581573\t0.963631\t9.883100\t-0.062090\t-0.048890\t52.124077\t0.000000\t0.000000\n\t\n15:05:03.1\tlog_raw\tgps_raw\t#INSPVAXA,USB3,0,46.0,FINESTEERING,2107,281120.450,02000000,471d,15824;INS_ALIGNMENT_COMPLETE,INS_RTKFIXED,37.37013887949,126.72084165446,9.8834,22.3000,0.0019,-0.0021,0.0014,-0.061789889,-0.048085749,35.914956839,0.1979,0.1659,0.2630,0.0381,0.0380,0.0312,0.3289,0.3384,5.3628,0f000015,0*c67f80b5\n\tsystem status\tnormal 0 28.400000 0 0\trobot status\t0.580132\t0.963677\t9.883400\t-0.061790\t-0.048086\t52.213058\t0.000000\t0.000000\n\t\n15:05:03.6\tlog_raw\tgps_raw\t#INSPVAXA,USB3,0,43.0,FINESTEERING,2107,281121.250,02000000,471d,15824;INS_ALIGNMENT_COMPLETE,INS_RTKFIXED,37.37013888537,126.72084165013,9.8842,22.3000,0.0022,-0.0011,0.0021,-0.060549213,-0.049924225,35.920563405,0.1978,0.1657,0.2626,0.0381,0.0380,0.0312,0.3289,0.3385,5.3503,0f000015,0*0a80ea0c\n\tsystem status\tnormal 0 28.400000 0 0\trobot status\t0.579749\t0.964330\t9.884200\t-0.060549\t-0.049924\t52.075462\t0.000000\t0.000000\n\t\n15:05:04.1\tlog_raw\tgps_raw\t#INSPVAXA,USB3,0,44.0,FINESTEERING,2107,281122.100,02000000,471d,15824;INS_ALIGNMENT_COMPLETE,INS_RTKFIXED,37.37013888493,126.72084163921,9.8848,22.3000,0.0016,-0.0024,0.0023,-0.056178885,-0.051797871,35.927971426,0.1977,0.1653,0.2621,0.0381,0.0380,0.0312,0.3289,0.3385,5.3378,0f000015,0*84da5f34\n\tsystem status\tnormal 0 28.400000 0 0\trobot status\t0.578782\t0.964281\t9.884800\t-0.056179\t-0.051798\t52.108948\t0.000000\t0.000000\n\t\n15:05:04.6\tlog_raw\tgps_raw\t#INSPVAXA,USB3,0,44.0,FINESTEERING,2107,281122.600,02000000,471d,15824;INS_ALIGNMENT_COMPLETE,INS_RTKFIXED,37.37013888307,126.72084163636,9.8851,22.3000,0.0018,-0.0018,0.0025,-0.054444541,-0.052377015,35.931430890,0.1977,0.1653,0.2621,0.0381,0.0380,0.0312,0.3289,0.3385,5.3378,0f000015,0*6c45dde3\n\tsystem status\tnormal 0 28.400000 0 0\trobot status\t0.578529\t0.964074\t9.885100\t-0.054445\t-0.052377\t52.230434\t0.000000\t-0.001000\n\t\n15:05:05.1\tlog_raw\tgps_raw\t#INSPVAXA,USB3,0,44.0,FINESTEERING,2107,281123.100,02000000,471d,15824;INS_ALIGNMENT_COMPLETE,INS_RTKFIXED,37.37013888356,126.72084163424,9.8854,22.3000,0.0020,-0.0003,0.0024,-0.054057362,-0.054517643,35.933045460,0.1976,0.1649,0.2616,0.0381,0.0380,0.0312,0.3288,0.3384,5.3256,0f000015,0*a8eaef80\n\tsystem status\tnormal 0 28.400000 0 0\trobot status\t0.578341\t0.964129\t9.885400\t-0.054057\t-0.054518\t52.035851\t0.000000\t0.000000\n\t\n15:05:05.6\tlog_raw\tgps_raw\t#DUALANTENNAHEADINGA,USB3,0,44.0,FINESTEERING,2107,281123.600,02000000,d426,15824;SOL_COMPUTED,NARROW_INT,-1.000000000,37.653594971,-13.557800293,0.0,0.579351723,0.952880502,\"631T\",30,20,20,15,04,00,30,33*ac2d0a42\n\tsystem status\tnormal 0 28.400000 0 0\trobot status\t0.578286\t0.963726\t9.885300\t-0.054720\t-0.056898\t52.346405\t0.000000\t-0.001000\n\t\n15:05:06.1\tlog_raw\tgps_raw\t#INSPVAXA,USB3,0,47.0,FINESTEERING,2107,281124.100,02000000,471d,15824;INS_ALIGNMENT_COMPLETE,INS_RTKFIXED,37.37013887631,126.72084163081,9.8854,22.3000,0.0008,-0.0001,0.0021,-0.054579567,-0.055627501,35.940324139,0.1974,0.1646,0.2611,0.0381,0.0380,0.0312,0.3288,0.3384,5.3278,0f000005,0*adb1451f\n\tsystem status\tnormal 0 28.400000 0 0\trobot status\t0.578038\t0.963324\t9.885400\t-0.054580\t-0.055628\t51.958927\t0.000000\t0.000000\n\t\n15:05:06.6\tlog_raw\tgps_raw\t#INSPVAXA,USB3,0,47.0,FINESTEERING,2107,281124.600,02000000,471d,15824;INS_ALIGNMENT_COMPLETE,INS_RTKFIXED,37.37013887904,126.72084162543,9.8852,22.3000,0.0018,-0.0013,0.0020,-0.055934568,-0.056307222,35.939178420,0.1974,0.1646,0.2611,0.0381,0.0380,0.0312,0.3288,0.3384,5.3278,0f000005,0*ea03628f\n\tsystem status\tnormal 0 28.400000 0 0\trobot status\t0.577561\t0.963627\t9.885200\t-0.055935\t-0.056307\t52.290703\t0.000000\t0.000000\n\t\n15:05:07.1\tlog_raw\tgps_raw\t#DUALANTENNAHEADINGA,USB3,0,43.0,FINESTEERING,2107,281125.100,02000000,d426,15824;SOL_COMPUTED,NARROW_INT,-1.000000000,37.642917633,-13.834228516,0.0,0.597326040,0.994234800,\"631T\",28,18,18,14,04,00,30,33*9c1b1646\n\tsystem status\tnormal 0 28.400000 0 0\trobot status\t0.576740\t0.964007\t9.885300\t-0.057114\t-0.057843\t52.357082\t0.000000\t0.000000\n\t\n15:05:07.6\tlog_raw\tgps_raw\t#INSPVAXA,USB3,0,43.0,FINESTEERING,2107,281125.600,02000000,471d,15824;INS_ALIGNMENT_COMPLETE,INS_RTKFIXED,37.37013888441,126.72084161551,9.8854,22.3000,0.0019,-0.0017,0.0024,-0.057645932,-0.058967433,35.933524606,0.1973,0.1645,0.2607,0.0381,0.0380,0.0312,0.3288,0.3384,5.3300,0f000005,0*b0b03c17\n\tsystem status\tnormal 0 28.400000 0 0\trobot status\t0.576682\t0.964223\t9.885400\t-0.057646\t-0.058967\t52.188740\t0.000000\t-0.001000\n\t\n15:05:08.1\tlog_raw\tgps_raw\t#DUALANTENNAHEADINGA,USB3,0,42.5,FINESTEERING,2107,281126.100,02000000,d426,15824;SOL_COMPUTED,NARROW_INT,-1.000000000,37.706222534,-13.263671875,0.0,0.593537927,0.794390440,\"631T\",29,18,18,14,04,00,30,33*6f53d1bd\n\tsystem status\tnormal 0 28.400000 0 0\trobot status\t0.576492\t0.964684\t9.885700\t-0.056417\t-0.058786\t52.293777\t0.000000\t-0.001000\n\t\n15:05:08.6\tlog_raw\tgps_raw\t#DUALANTENNAHEADINGA,USB3,0,42.5,FINESTEERING,2107,281126.600,02000000,d426,15824;SOL_COMPUTED,NARROW_INT,-1.000000000,37.709869385,-13.478881836,0.0,0.638457775,0.856098652,\"631T\",30,18,18,14,04,00,30,33*210d1ede\n\tsystem status\tnormal 0 28.400000 0 0\trobot status\t0.576413\t0.964629\t9.885600\t-0.055415\t-0.061255\t52.290131\t0.000000\t-0.001000\n\t\n15:05:09.1\tlog_raw\tgps_raw\t#DUALANTENNAHEADINGA,USB3,0,41.5,FINESTEERING,2107,281127.100,02000000,d426,15824;SOL_COMPUTED,NARROW_INT,-1.000000000,37.626621246,-14.364105225,0.0,0.640958905,0.860277176,\"631T\",28,18,18,13,04,00,30,33*f099c15c\n\tsystem status\tnormal 0 28.300000 0 0\trobot status\t0.576518\t0.964884\t9.885800\t-0.055656\t-0.061223\t52.373379\t0.000000\t0.000000\n\t\n15:05:09.6\tlog_raw\tgps_raw\t#DUALANTENNAHEADINGA,USB3,0,41.5,FINESTEERING,2107,281127.600,02000000,d426,15824;SOL_COMPUTED,NARROW_INT,-1.000000000,37.695549011,-13.609527588,0.0,0.638991773,0.872274935,\"631T\",29,18,18,13,04,00,30,33*cb6ad9c8\n\tsystem status\tnormal 0 28.400000 0 0\trobot status\t0.576518\t0.964987\t9.886000\t-0.056146\t-0.060371\t52.304451\t0.000000\t0.000000\n\t\n15:05:10.1\tlog_raw\tgps_raw\t#DUALANTENNAHEADINGA,USB3,0,40.5,FINESTEERING,2107,281128.100,02000000,d426,15824;SOL_COMPUTED,NARROW_INT,-1.000000000,37.677280426,-12.618164063,0.0,0.634656608,0.868122041,\"631T\",31,18,18,13,04,00,30,33*cb4c8f66\n\tsystem status\tnormal 0 28.300000 0 0\trobot status\t0.576086\t0.965186\t9.886100\t-0.055057\t-0.058970\t52.322720\t0.000000\t-0.001000\n\t\n15:05:10.6\tlog_raw\tgps_raw\t#INSPVAXA,USB3,0,40.5,FINESTEERING,2107,281128.600,02000000,471d,15824;INS_ALIGNMENT_COMPLETE,INS_RTKFIXED,37.37013889265,126.72084160793,9.8862,22.3000,0.0022,-0.0007,0.0017,-0.055232620,-0.058016888,35.929747636,0.1969,0.1638,0.2593,0.0381,0.0381,0.0312,0.3287,0.3383,5.3366,0f000005,0*7a2477b1\n\tsystem status\tnormal 0 28.400000 0 0\trobot status\t0.576011\t0.965138\t9.886200\t-0.055233\t-0.058017\t51.759930\t0.000000\t-0.001000\n\t\n15:05:11.1\tlog_raw\tgps_raw\t#DUALANTENNAHEADINGA,USB3,0,40.5,FINESTEERING,2107,281129.100,02000000,d426,15824;SOL_COMPUTED,NARROW_INT,-1.000000000,38.138561249,-13.762512207,0.0,0.610144854,0.795504868,\"631T\",29,18,18,13,04,00,30,33*c71c4996\n\tsystem status\tnormal 0 28.400000 0 0\trobot status\t0.575878\t0.965334\t9.886300\t-0.056356\t-0.060093\t51.861439\t0.000000\t-0.001000\n\t\n15:05:11.6\tlog_raw\tgps_raw\t#DUALANTENNAHEADINGA,USB3,0,45.0,FINESTEERING,2107,281129.600,02000000,d426,15824;SOL_COMPUTED,NARROW_INT,-1.000000000,37.785083771,-12.632385254,0.0,0.627400696,0.824337482,\"631T\",29,19,19,14,04,00,30,33*31b2c303\n\tsystem status\tnormal 0 28.400000 0 0\trobot status\t0.575575\t0.965088\t9.886100\t-0.056551\t-0.060488\t52.214916\t0.000000\t0.000000\n\t\n15:05:12.1\tlog_raw\tgps_raw\t#INSPVAXA,USB3,0,45.0,FINESTEERING,2107,281130.100,02000000,471d,15824;INS_ALIGNMENT_COMPLETE,INS_RTKFIXED,37.37013889099,126.72084159619,9.8861,22.3000,0.0016,-0.0021,0.0019,-0.057319061,-0.062128456,35.918616940,0.1967,0.1636,0.2585,0.0381,0.0380,0.0312,0.3286,0.3381,5.3411,0f000005,0*4275ce6a\n\tsystem status\tnormal 0 28.400000 0 0\trobot status\t0.574971\t0.964953\t9.886100\t-0.057319\t-0.062128\t52.123562\t0.000000\t0.000000\n\t\n15:05:12.6\tlog_raw\tgps_raw\t#INSPVAXA,USB3,0,46.0,FINESTEERING,2107,281130.600,02000000,471d,15824;INS_ALIGNMENT_COMPLETE,INS_RTKFIXED,37.37013889026,126.72084159618,9.8864,22.3000,0.0023,-0.0018,0.0019,-0.055730148,-0.062639805,35.917950244,0.1967,0.1636,0.2585,0.0381,0.0380,0.0312,0.3286,0.3381,5.3411,0f000005,0*68e0adb8\n\tsystem status\tnormal 0 28.400000 0 0\trobot status\t0.574970\t0.964872\t9.886400\t-0.055730\t-0.062640\t52.461452\t0.000000\t-0.001000\n\t\n15:05:13.1\tlog_raw\tgps_raw\t#DUALANTENNAHEADINGA,USB3,0,45.5,FINESTEERING,2107,281131.100,02000000,d426,15824;SOL_COMPUTED,NARROW_INT,-1.000000000,37.898468018,-13.103790283,0.0,0.640745819,0.864472210,\"631T\",28,19,19,15,04,00,30,33*c85a74f5\n\tsystem status\tnormal 0 28.400000 0 0\trobot status\t0.574928\t0.965170\t9.886800\t-0.053563\t-0.061883\t52.101532\t0.000000\t-0.001000\n\t\n15:05:13.6\tlog_raw\tgps_raw\t#DUALANTENNAHEADINGA,USB3,0,45.5,FINESTEERING,2107,281131.600,02000000,d426,15824;SOL_COMPUTED,NARROW_INT,-1.000000000,37.923900604,-13.462554932,0.0,0.777255595,1.286689639,\"631T\",29,20,20,15,04,00,30,33*b16e5ca0\n\tsystem status\tnormal 0 28.400000 0 0\trobot status\t0.574668\t0.965413\t9.886900\t-0.051217\t-0.062505\t52.076099\t0.000000\t-0.001000\n\t\n15:05:14.1\tlog_raw\tgps_raw\t#DUALANTENNAHEADINGA,USB3,0,43.0,FINESTEERING,2107,281132.100,02000000,d426,15824;SOL_COMPUTED,NARROW_INT,-1.000000000,38.050197601,-14.205993652,0.0,0.752799392,1.190752268,\"631T\",29,20,20,15,04,00,30,33*d9e48ae9\n\tsystem status\tnormal 0 28.400000 0 0\trobot status\t0.574463\t0.965930\t9.887000\t-0.051518\t-0.061857\t51.949802\t0.000000\t0.000000\n\t\n15:05:14.6\tlog_raw\tgps_raw\t#DUALANTENNAHEADINGA,USB3,0,43.0,FINESTEERING,2107,281132.600,02000000,d426,15824;SOL_COMPUTED,NARROW_INT,-1.000000000,38.002994537,-14.216644287,0.0,0.630166113,1.172435641,\"631T\",27,20,20,14,04,00,30,33*17fcf534\n\tsystem status\tnormal 0 28.400000 0 0\trobot status\t0.574327\t0.965726\t9.887000\t-0.049713\t-0.061845\t51.997005\t0.000000\t-0.001000\n\t\n15:05:15.1\tlog_raw\tgps_raw\t#INSPVAXA,USB3,0,44.5,FINESTEERING,2107,281133.100,02000000,471d,15824;INS_ALIGNMENT_COMPLETE,INS_RTKFIXED,37.37013889858,126.72084158985,9.8870,22.3000,0.0026,-0.0001,0.0019,-0.047158165,-0.062046751,35.902498944,0.1965,0.1632,0.2574,0.0381,0.0380,0.0312,0.3286,0.3381,5.3478,0f000005,0*267c8665\n\tsystem status\tnormal 0 28.400000 0 0\trobot status\t0.574409\t0.965796\t9.887000\t-0.047158\t-0.062047\t52.045242\t0.000000\t-0.001000\n\t\n15:05:15.6\tlog_raw\tgps_raw\t#DUALANTENNAHEADINGA,USB3,0,44.5,FINESTEERING,2107,281133.600,02000000,d426,15824;SOL_COMPUTED,NARROW_INT,-1.000000000,37.266918182,-13.973144531,0.0,0.960284948,1.937353253,\"631T\",29,18,18,14,04,00,30,33*dbf1b9cc\n\tsystem status\tnormal 0 28.400000 0 0\trobot status\t0.574679\t0.965706\t9.887300\t-0.047268\t-0.060593\t52.733082\t0.000000\t-0.001000\n\t\n15:05:16.1\tlog_raw\tgps_raw\t#INSPVAXA,USB3,0,41.5,FINESTEERING,2107,281134.100,02000000,471d,15824;INS_ALIGNMENT_COMPLETE,INS_RTKFIXED,37.37013889971,126.72084160146,9.8878,22.3000,0.0027,0.0022,0.0027,-0.046373760,-0.059690361,35.894790121,0.1968,0.1641,0.2580,0.0381,0.0381,0.0312,0.3283,0.3378,5.3500,0f000005,0*e92be400\n\tsystem status\tnormal 0 28.400000 0 0\trobot status\t0.575438\t0.965921\t9.887800\t-0.046374\t-0.059690\t52.569603\t0.000000\t-0.001000\n\t\n15:05:16.6\tlog_raw\tgps_raw\t#DUALANTENNAHEADINGA,USB3,0,41.5,FINESTEERING,2107,281134.600,02000000,d426,15824;SOL_COMPUTED,NARROW_INT,-1.000000000,37.776412964,-12.936340332,0.0,0.785194933,1.219629526,\"631T\",28,18,18,14,04,00,30,33*9fa2cd7d\n\tsystem status\tnormal 0 28.400000 0 0\trobot status\t0.575432\t0.965903\t9.887700\t-0.045093\t-0.057079\t52.223587\t0.000000\t0.000000\n\t\n15:05:17.1\tlog_raw\tgps_raw\t#INSPVAXA,USB3,0,41.5,FINESTEERING,2107,281135.100,02000000,471d,15824;INS_ALIGNMENT_COMPLETE,INS_RTKFIXED,37.37013889960,126.72084160417,9.8880,22.3000,0.0014,0.0025,0.0032,-0.044104589,-0.053679720,35.890980507,0.1970,0.1649,0.2586,0.0381,0.0380,0.0312,0.3283,0.3378,5.3522,0f000005,0*afe9f7e8\n\tsystem status\tnormal 0 28.300000 0 0\trobot status\t0.575678\t0.965909\t9.888000\t-0.044105\t-0.053680\t51.956696\t0.000000\t0.000000\n\t\n15:05:17.6\tlog_raw\tgps_raw\t#DUALANTENNAHEADINGA,USB3,0,46.5,FINESTEERING,2107,281135.600,02000000,d426,15824;SOL_COMPUTED,NARROW_INT,-1.000000000,38.299953461,-12.993041992,0.0,0.993980289,1.004105210,\"631T\",25,14,14,10,04,00,10,33*25d1fb28\n\tsystem status\tnormal 0 28.300000 0 0\trobot status\t0.575508\t0.965479\t9.888200\t-0.042354\t-0.052670\t51.700047\t0.000000\t0.000000\n\t\n15:05:18.1\tlog_raw\tgps_raw\t#DUALANTENNAHEADINGA,USB3,0,46.5,FINESTEERING,2107,281136.100,02000000,d426,15824;SOL_COMPUTED,NARROW_INT,-1.000000000,38.161273956,-12.752471924,0.0,1.404599905,1.380629778,\"631T\",27,14,14,10,04,00,10,33*6d978cd4\n\tsystem status\tnormal 0 28.300000 0 0\trobot status\t0.575378\t0.964929\t9.888600\t-0.043547\t-0.050957\t51.838726\t0.000000\t-0.001000\n\t\n15:05:18.6\tlog_raw\tgps_raw\t#DUALANTENNAHEADINGA,USB3,0,47.5,FINESTEERING,2107,281136.600,02000000,d426,15824;SOL_COMPUTED,NARROW_INT,-1.000000000,38.175228119,-13.140533447,0.0,1.065542459,1.250077486,\"631T\",26,18,18,14,04,00,30,33*16ca9040\n\tsystem status\tnormal 0 28.400000 0 0\trobot status\t0.575286\t0.964698\t9.888400\t-0.043927\t-0.049967\t51.824772\t0.000000\t-0.001000\n\t\n15:05:19.1\tlog_raw\tgps_raw\t#DUALANTENNAHEADINGA,USB3,0,44.0,FINESTEERING,2107,281137.100,02000000,d426,15824;SOL_COMPUTED,NARROW_INT,-1.000000000,38.409736633,-12.959808350,0.0,0.979367137,1.144175768,\"631T\",26,18,18,14,04,00,30,33*dc594a4a\n\tsystem status\tnormal 0 28.400000 0 0\trobot status\t0.575437\t0.964386\t9.888200\t-0.044307\t-0.050467\t51.590263\t0.000000\t0.000000\n\t\n15:05:19.6\tlog_raw\tgps_raw\t#DUALANTENNAHEADINGA,USB3,0,44.0,FINESTEERING,2107,281137.600,02000000,d426,15824;SOL_COMPUTED,NARROW_INT,-1.000000000,38.120170593,-13.114624023,0.0,0.905129552,1.058885336,\"631T\",25,18,18,14,04,00,30,23*290e79b4\n\tsystem status\tnormal 0 28.400000 0 0\trobot status\t0.575363\t0.964125\t9.887700\t-0.045017\t-0.050492\t51.879829\t0.000000\t0.000000\n\t\n15:05:20.1\tlog_raw\tgps_raw\t#DUALANTENNAHEADINGA,USB3,0,44.0,FINESTEERING,2107,281138.100,02000000,d426,15824;SOL_COMPUTED,NARROW_INT,-1.000000000,38.179969788,-13.311553955,0.0,0.848227024,1.002028346,\"631T\",25,18,18,14,04,00,30,23*9d9d193b\n\tsystem status\tnormal 0 28.400000 0 0\trobot status\t0.575695\t0.963721\t9.887300\t-0.045947\t-0.048789\t51.820030\t0.000000\t0.000000\n\t\n15:05:20.6\tlog_raw\tgps_raw\t#DUALANTENNAHEADINGA,USB3,0,46.5,FINESTEERING,2107,281138.600,02000000,d426,15824;SOL_COMPUTED,NARROW_INT,-1.000000000,38.178440094,-12.544708252,0.0,1.232779741,1.512524366,\"631T\",24,14,14,13,04,00,20,23*fc27c74c\n\tsystem status\tnormal 0 28.400000 0 0\trobot status\t0.576191\t0.963367\t9.887200\t-0.045548\t-0.049190\t51.821560\t0.000000\t-0.001000\n\t\n15:05:21.1\tlog_raw\tgps_raw\t#DUALANTENNAHEADINGA,USB3,0,46.5,FINESTEERING,2107,281139.100,02000000,d426,15824;SOL_COMPUTED,NARROW_INT,-1.000000000,37.941974640,-12.764343262,0.0,1.180174351,1.434758425,\"631T\",23,14,14,13,04,00,30,33*df4e4064\n\tsystem status\tnormal 0 28.400000 0 0\trobot status\t0.577135\t0.963101\t9.887400\t-0.045465\t-0.049701\t52.058025\t0.000000\t-0.001000\n\t\n15:05:21.6\tlog_raw\tgps_raw\t\tsystem status\tnormal 0 28.400000 0 0\trobot status\t0.576914\t0.962846\t9.886700\t-0.045050\t-0.049482\t52.393593\t0.000000\t0.000000\n\t\n15:05:22.1\tlog_raw\tgps_raw\t#DUALANTENNAHEADINGA,USB3,0,46.5,FINESTEERING,2107,281140.100,02000000,d426,15824;SOL_COMPUTED,NARROW_INT,
